vi "还原为字符串.vi"(8 "error in (no error)":errorcluster caption="错误输入（无错误）", 10 "输入数组":u16[](array[numeric])) -> (0 "error out":errorcluster caption="错误输出", 2 "字符串":string)   [LabVIEW 2018]
panel:
  out "数组":u16[](array[numeric])
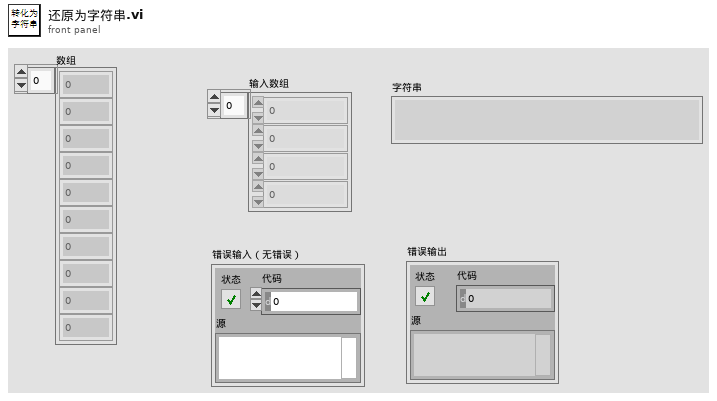
[diagram p1: front panel]
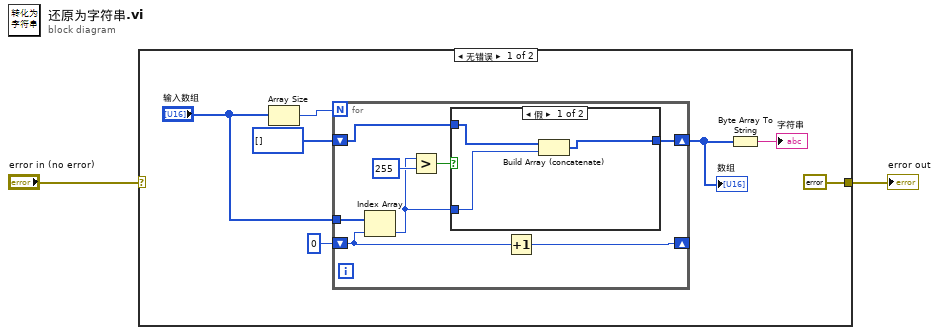
[diagram p0: block diagram]
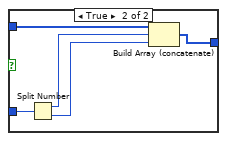
[diagram p2: hidden frame]
diagram:
  n1 = case shown="无错误" "error in (no error)" {
    selector: "error in (no error)" -> [_ w26]
    tunnel: [errorcluster {"status"=FALSE, "code"=0, "source"=""} ("error IO") w26] -> w1
    frame No Error {
      n2 = Array Size(array="输入数组") -> (size(s)=w6:i32)
      n3 = for {
        N: w6 -> [_]
        shift-right: [w16] -> _
        shift-left: 0 -> [w17]
        shift-right: [w15] -> w4
        shift-left: u8[] [] -> [w14]
        tunnel: "输入数组" -> [w13]
        n4 = Index Array(array=w13, index=w17) -> (element=w10:u16)
        n5 = Greater?(x=w10, y=u16 255) -> (0:w12:bool)
        n6 = case shown="假" w12 {
          tunnel: [w18 w25] -> w15
          tunnel: w14 -> [w20 w24]
          tunnel: w10 -> [w19 w21]
          frame False {
            n7 = Build Array (concatenate)(w20, w19) -> (w18:u16[])
          }
          frame True {
            n8 = Split Number(x=w21) -> (hi(x)=w23:u8, lo(x)=w22:u8)
            n9 = Build Array (concatenate)(w24, w23, w22) -> (w25:u16[])
          }
        }
        n10 = Increment(x=w17) -> (x+1=w16:i32)
      }
      "数组" <- w4
      n11 = Byte Array To String(unsigned byte array=w4) -> (string=→"字符串":string)
    }
    frame Error {
    }
  }
  "error out" <- w1
